vi "WilliamsEncoder.vi"(9 "Delta T":dbl=100.0, 10 "Distance 2":dbl, 11 "Distance 1":dbl) -> (2 "Rate 2":dbl, 3 "Rate 1":dbl)   [LabVIEW 2015]
panel:
  out "Time elapsed":u64
  in  "Instance":dbl
  in  "old Dist 2 (2)":dbl
  in  "old Dist 1 (2)":dbl
  in  "old Dist 2 (1)":dbl
  in  "old Dist 1 (1)":dbl
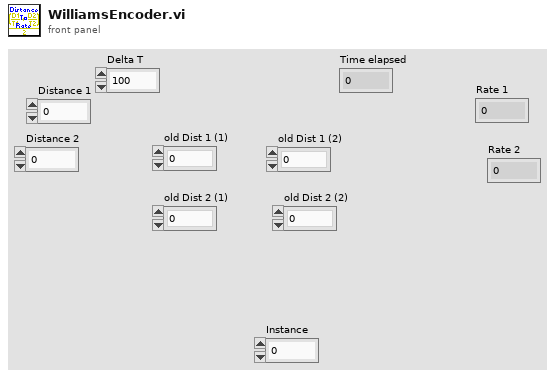
[diagram p1: front panel]
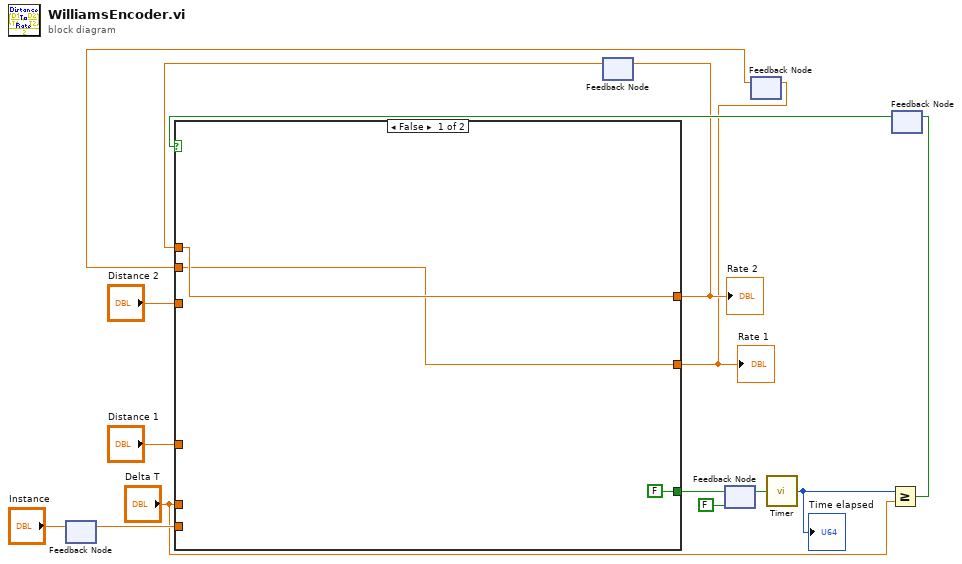
[diagram p0: block diagram]
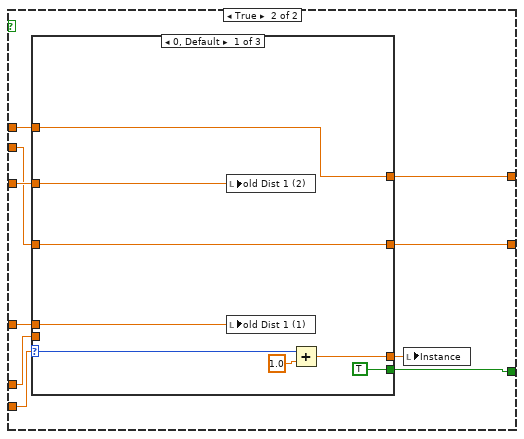
[diagram p2: hidden frame]
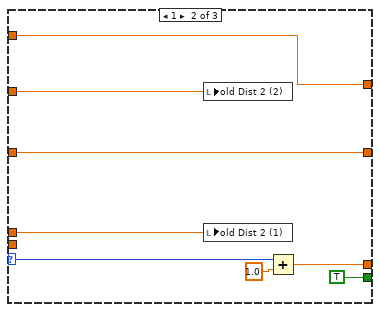
[diagram p3: hidden frame]
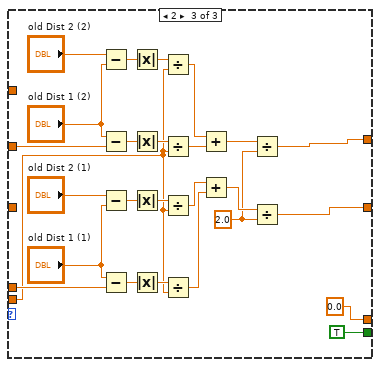
[diagram p4: hidden frame]
diagram:
  n1 = feedback #1() -> (w11:dbl)  [unwired: 1 in]
  n2 = feedback-in #1("Instance") -> ()
  n3 = feedback #2() -> (w3:dbl)  [unwired: 1 in]
  n4 = feedback #3(FALSE) -> (w9:bool)
  n5 = feedback #4() -> (w1:dbl)  [unwired: 1 in]
  n6 = call "Timer.vi"("Start Timer"=w9) -> ("Time elapsed"=w15:u64)
  "Time elapsed" <- w15
  n7 = Greater Or Equal?(x=w15, y="Delta T") -> (x >= y?=w14:bool)
  n8 = feedback #5() -> (w13:bool)  [unwired: 1 in]
  n9 = case shown="False" w13 {
    tunnel: w11 -> [_ w28]
    tunnel: [FALSE w27] -> w10
    tunnel: "Distance 1" -> [_ w25]
    tunnel: "Distance 2" -> [_ w24]
    tunnel: "Delta T" -> [_ w23]
    tunnel: [w17 w22] -> w4
    tunnel: [w16 w21] -> w2
    tunnel: w3 -> [w17 w20]
    tunnel: w1 -> [w16 w19]
    frame False {
    }
    frame True {
      n10 = case shown="0, Default" w28 {
        selector: w28 -> [w35 w44 _]
        tunnel: [TRUE TRUE TRUE] -> w27
        tunnel: [w34 w42 0.0 ("y")] -> w26
        tunnel: w25 -> [w32 w39 w56]
        tunnel: w24 -> [w31 w40 w64]
        tunnel: w23 -> [_ _ w51]
        tunnel: [w30 w38 w46] -> w22
        tunnel: [w29 w37 w45] -> w21
        tunnel: w20 -> [w30 w38 _]
        tunnel: w19 -> [w29 w37 _]
        frame 0, Default {
          n11 = local write "old Dist 1 (2)"(w31) -> ()
          n12 = local write "old Dist 1 (1)"(w32) -> ()
          n13 = Add(x=w35, y=1.0) -> (x+y=w34:dbl)
        }
        frame 1 {
          n14 = local write "old Dist 2 (2)"(w40) -> ()
          n15 = local write "old Dist 2 (1)"(w39) -> ()
          n16 = Add(x=w44, y=1.0) -> (x+y=w42:dbl)
        }
        frame 2 {
          w47 = 2.0 ("y")
          n17 = Subtract(x="old Dist 2 (2)", y="old Dist 1 (2)") -> (x-y=w67:dbl)
          n18 = Subtract(x="old Dist 1 (2)", y=w64) -> (x-y=w63:dbl)
          n19 = Subtract(x="old Dist 2 (1)", y="old Dist 1 (1)") -> (x-y=w55:dbl)
          n20 = Subtract(x="old Dist 1 (1)", y=w56) -> (x-y=w53:dbl)
          n21 = Absolute Value(x=w67) -> (abs(x)=w66:dbl)
          n22 = Absolute Value(x=w63) -> (abs(x)=w62:dbl)
          n23 = Absolute Value(x=w55) -> (abs(x)=w54:dbl)
          n24 = Absolute Value(x=w53) -> (abs(x)=w52:dbl)
          n25 = Divide(x=w66, y=w51) -> (x/y=w61:dbl)
          n26 = Divide(x=w62, y=w51) -> (x/y=w60:dbl)
          n27 = Divide(x=w54, y=w51) -> (x/y=w50:dbl)
          n28 = Divide(x=w52, y=w51) -> (x/y=w49:dbl)
          n29 = Add(x=w61, y=w60) -> (x+y=w59:dbl)
          n30 = Add(x=w50, y=w49) -> (x+y=w48:dbl)
          n31 = Divide(x=w59, y=w47) -> (x/y=w46:dbl)
          n32 = Divide(x=w48, y=w47) -> (x/y=w45:dbl)
        }
      }
      n33 = local write "Instance"(w26) -> ()
    }
  }
  "Rate 1" <- w2
  "Rate 2" <- w4
  n34 = feedback-in #2(w4) -> ()
  n35 = feedback-in #3(w10) -> ()
  n36 = feedback-in #4(w2) -> ()
  n37 = feedback-in #5(w14) -> ()
